vi "Teleop.vi"(10 "Match Info":T1={"Autonomous Elapsed Seconds"=0.0, "TeleOp Elapsed Seconds"=0.0, "Disabled Elapsed Seconds"=0.0, "Visited Autonomous"=FALSE, "Visited TeleOp"=FALSE, "Visited Disabled"=FALSE, "Autonomous Settings"={"Autonomous Style"=enum."Independent", "VI Refnum"=refnum}}, 11 "Call Context":T2) -> ()   [LabVIEW 2018]
doc: "This VI is called for each TeleOp packet received from the DS where the robot is not disabled. It is often used to read from the joysticks and update I/O or to update setpoints for timed control loops. It should complete and return within 20 milliseconds or it may miss DS packets."
uses:
  <vilib>/Rock Robotics/WPI/DriverStation/WPI_DriverStationDerivedRobotMode.ctl
  <vilib>/Rock Robotics/WPI/DriverStation/WPI_DriverStationMatch Info.ctl
  <vilib>/Rock Robotics/Network Tables/NT Read Boolean.vi
  <vilib>/Rock Robotics/Network Tables/NT Read Number.vi
  <vilib>/Rock Robotics/WPI/Utilities/WPI_GetSetVariantRefNum.vi
  <vilib>/Rock Robotics/Network Tables/NT Write Boolean Array.vi
  <vilib>/Rock Robotics/Network Tables/NT Write Numeric Array.vi
  <vilib>/Rock Robotics/Network Tables/NT Read Numeric Array.vi
  <vilib>/Rock Robotics/Network Tables/NT Write Boolean.vi
  <vilib>/Rock Robotics/Network Tables/NT Write Number.vi
panel:
  in  "Motor Stall":dbl format="%#_13g"
  out "Sample Slider 0":dbl(slide) scale=0.0..5.0
  out "Sample Boolean 1":bool
  out "Sample Boolean 0":bool
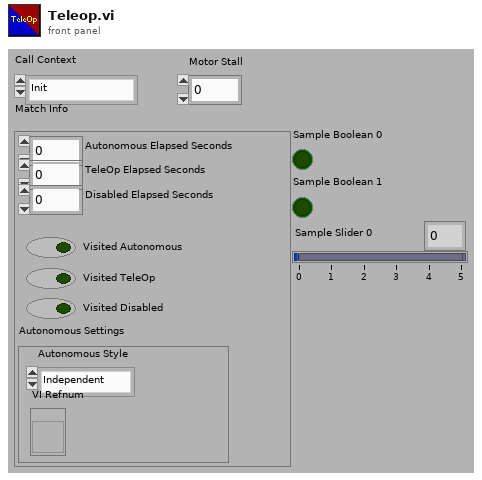
[diagram p1: front panel]
types:
  T1 = typedef "WPI_DriverStationMatch Info.ctl" = cluster{"Autonomous Elapsed Seconds":dbl, "TeleOp Elapsed Seconds":dbl, "Disabled Elapsed Seconds":dbl, "Visited Autonomous":bool, "Visited TeleOp":bool, "Visited Disabled":bool, "Autonomous Settings":cluster{"Autonomous Style":enum16{"Iterative", "Independent"}, "VI Refnum":refnum<vi>}}
  T2 = typedef "WPI_DriverStationDerivedRobotMode.ctl" = enum16{"Init", "Execute", "Stop"}
  T3 = typedef "WPI_JoystickDevRef.ctl" = cluster{"Device":T4}
  T4 = typedef "WPI_JoystickDeviceEnum.ctl" = enum16{"USB 0", "USB 1", "USB 2", "USB 3", "USB 4", "USB 5"}
  T5 = typedef "WPI_MotorControlDeviceRef.ctl" = cluster{"DeviceStatus":errorcluster, "Type":T6, "PWM":cluster{"PWM Channel":T7, "DeadBand":T8}, "CAN":cluster{"Device Number":u8, "SetOutput VI Ref":variant, "GetOutput VI Ref":variant, "Enable VI Ref":variant, "Disable VI Ref":variant, "Data":variant}, "Invert":bool, "DIO PWM":cluster{"PWM \"Enable\" Channel":T7, "DIOChannel":T9, "PWM Rate":dbl}}
  T6 = typedef "WPI_MotorControlType.ctl" = enum16{"PWM", "CAN", "DIO PWM"}
  T7 = typedef "FPGA_DIOPWMChannel.ctl" = enum8{"PWM 0", "PWM 1", "PWM 2", "PWM 3", "PWM 4", "PWM 5", "PWM 6", "PWM 7", "PWM 8", "PWM 9", "PWM MXP 0", "PWM MXP 1", "PWM MXP 2", "PWM MXP 3", "PWM MXP 4", "PWM MXP 5", "PWM MXP 6", "PWM MXP 7", "PWM MXP 8", "PWM MXP 9", "Invalid"}
  T8 = typedef "WPI_PWMDeadband.ctl" = cluster{"Name":string, "maxPositivePwm":i32, "minPositivePwm":i32, "centerPwm":i32, "maxNegativePwm":i32, "minNegativePwm":i32, "angularRange":u16}
  T9 = typedef "FPGA_DIOChannel.ctl" = enum8{"DIO 0", "DIO 1", "DIO 2", "DIO 3", "DIO 4", "DIO 5", "DIO 6", "DIO 7", "DIO 8", "DIO 9", "DIO MXP 0", "DIO MXP 1", "DIO MXP 2", "DIO MXP 3", "DIO MXP 4", "DIO MXP 5", "DIO MXP 6", "DIO MXP 7", "DIO MXP 8", "DIO MXP 9", "DIO MXP 10", "DIO MXP 11", "DIO MXP 12", "DIO MXP 13", "DIO MXP 14", "DIO MXP 15", "SPI Port CS1", "SPI Port CS2", "SPI Port CS3", "SPI Port MISO", "SPI Port MOSI", "Invalid"}
  T10 = typedef "WPI_RobotDriveDevRef.ctl" = cluster{"DevStatus":errorcluster, "Motors[]":T5[], "Square Inputs":bool, "Max Output":dbl}
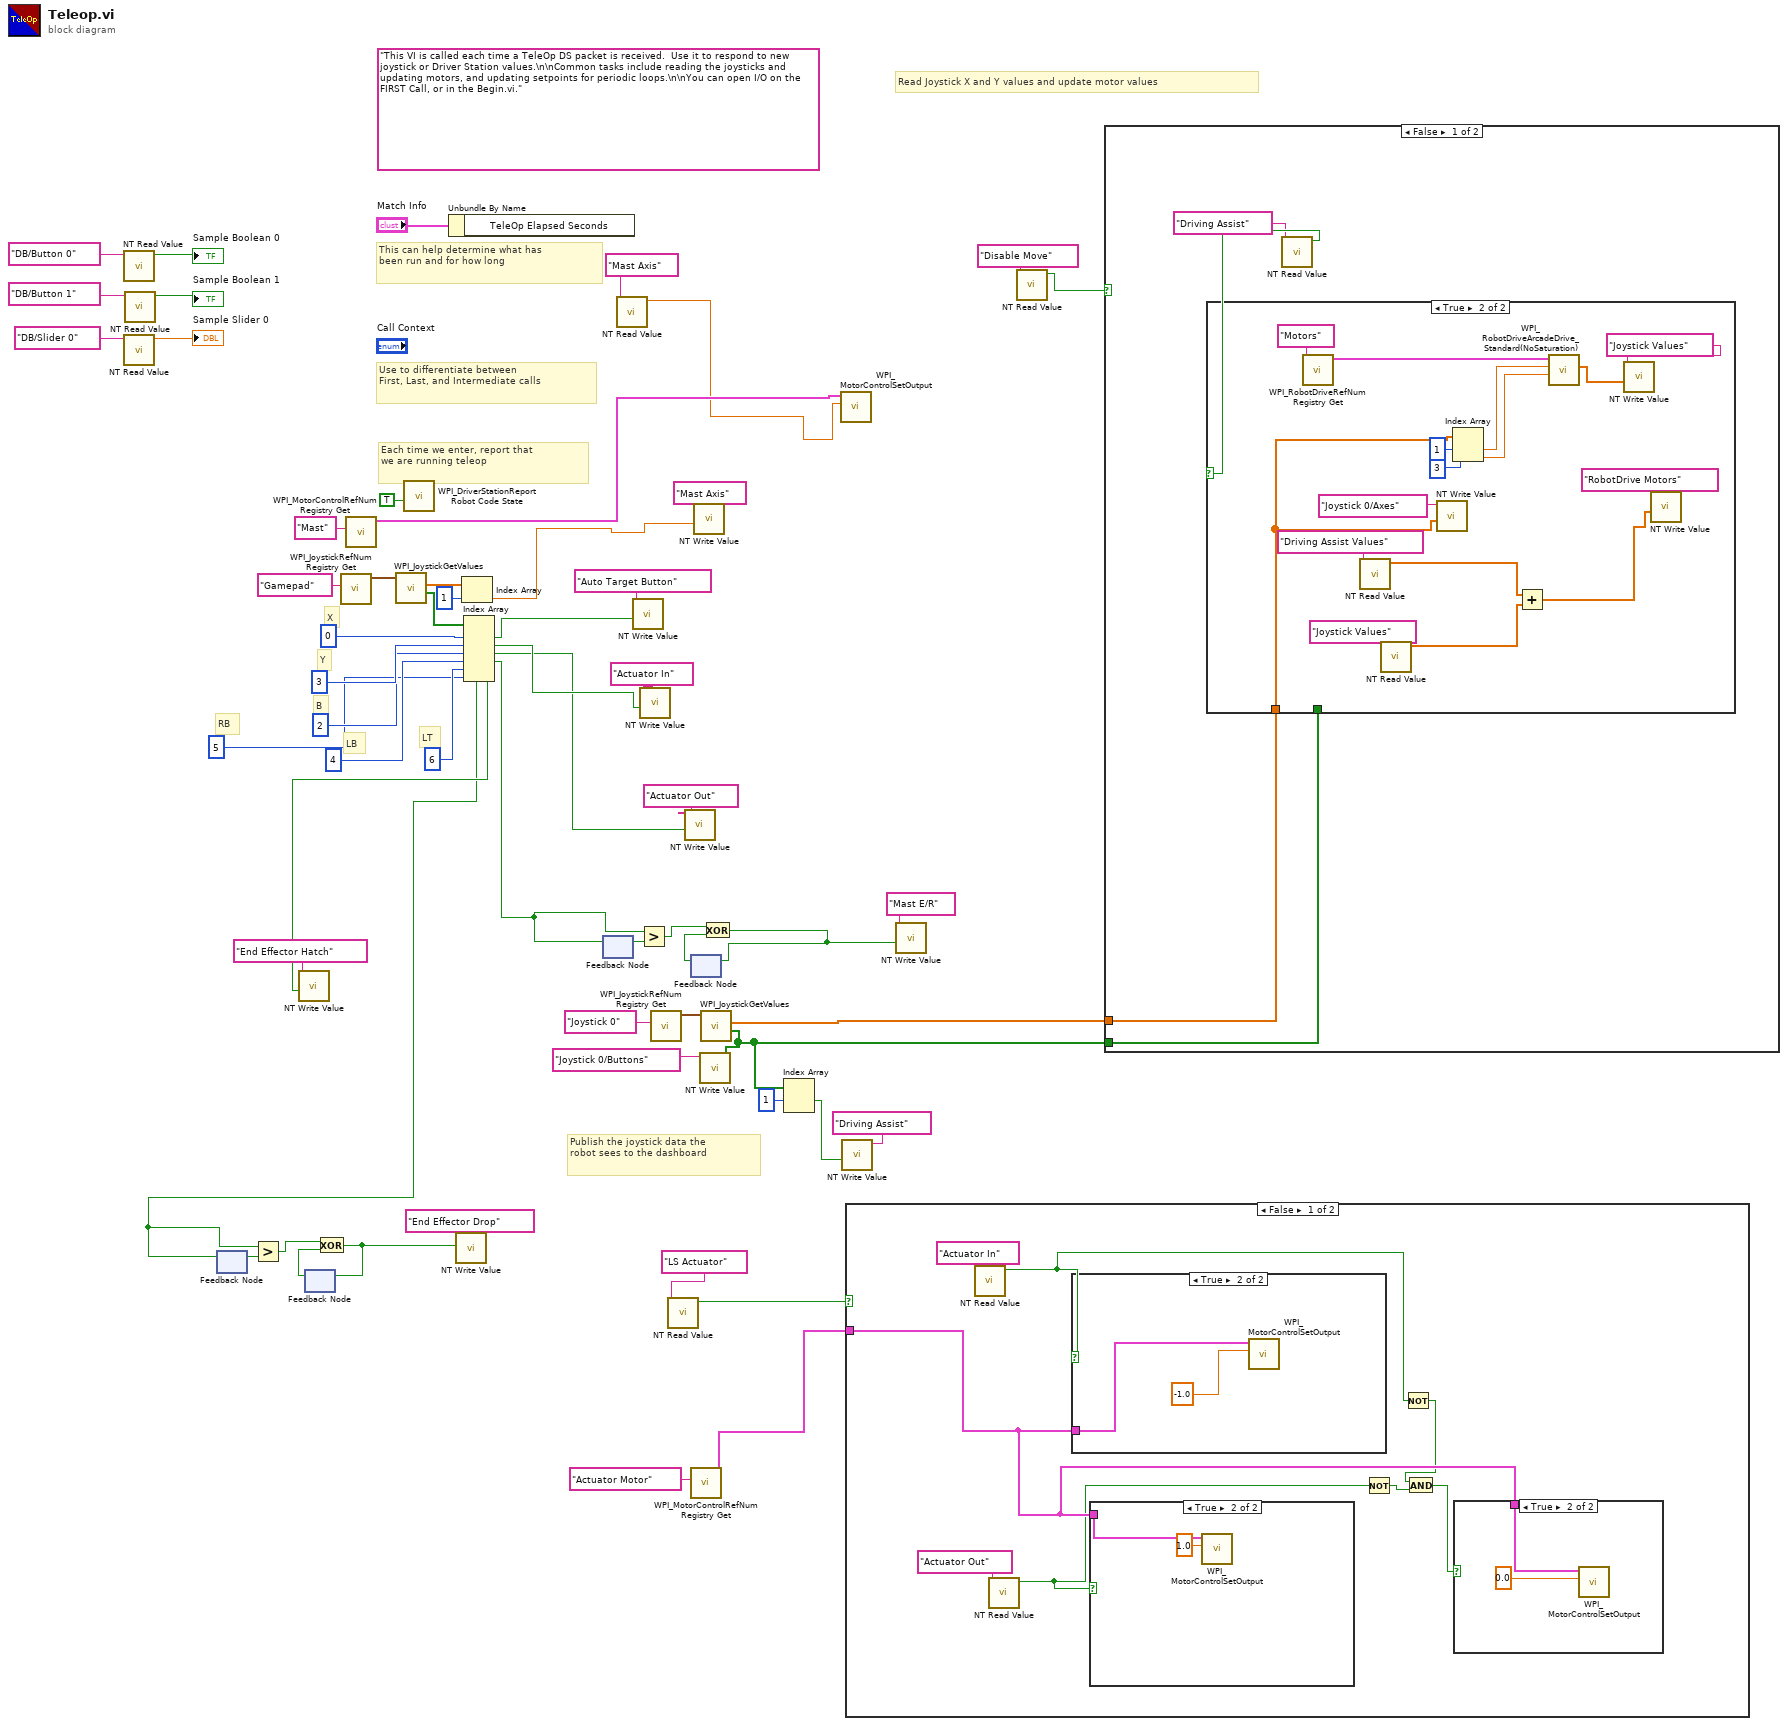
[diagram p0: block diagram]
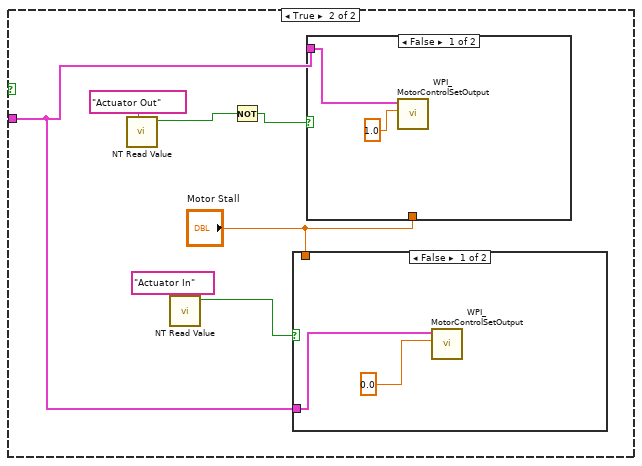
[diagram p5: hidden frame]
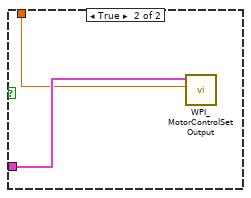
[diagram p6: hidden frame]
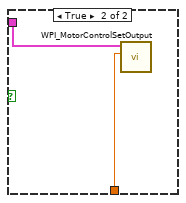
[diagram p7: hidden frame]
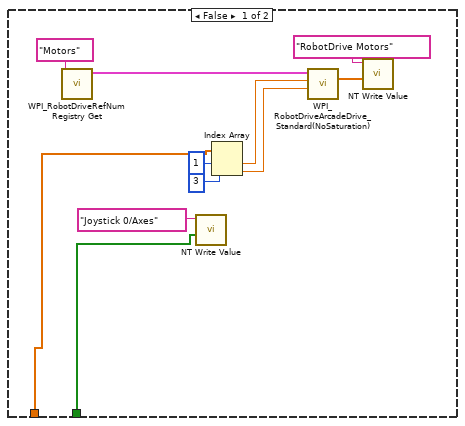
[diagram p8: hidden frame]
diagram:
  (unwired) "This VI is called each time a TeleOp DS packet is received.  Use it to respond to new joystick or Driver Station values.\n\nCommon tasks include reading the joysticks and updating motors, and updating setpoints for periodic loops.\n\nYou can open I/O on the FIRST Call, or in the Begin.vi."
  # "RB"
  # "LT"
  # "LB"
  # "Publish the joystick data the\nrobot sees to the dashboard"
  # "B"
  # "X"
  # "Y"
  # "Each time we enter, report that\nwe are running teleop"
  # "Use to differentiate between\nFirst, Last, and Intermediate calls"
  # "This can help determine what has\nbeen run and for how long"
  # "Read Joystick X and Y values and update motor values"
  n1 = call-poly <vilib>:"NT Read Value.vi"("Name"="DB/Button 0" ("refnum name")) -> ("Boolean"=→"Sample Boolean 0":bool)  [unwired: 9 in, 1 out]
  n2 = call-poly <vilib>:"NT Read Value.vi"("Name"="DB/Slider 0" ("refnum name")) -> ("Numeric"=→"Sample Slider 0":dbl)  [unwired: 9 in, 1 out]
  n3 = call-poly <vilib>:"NT Read Value.vi"("Name"="DB/Button 1" ("refnum name")) -> ("Boolean"=→"Sample Boolean 1":bool)  [unwired: 9 in, 1 out]
  n4 = feedback #1() -> (w5:bool)  [unwired: 1 in]
  n5 = feedback #2() -> (w3:bool)  [unwired: 1 in]
  n6 = call <vilib>:"WPI_JoystickRefNum Registry Get.vi"("refnum name"="Gamepad") -> ("JoystickDevRef"=w49:T3)  [unwired: 9 in, 1 out]
  n7 = call <vilib>:"WPI_MotorControlRefNum Registry Get.vi"("refnum name"="Mast") -> ("MotorControlDevRef"=w12:T5)  [unwired: 9 in, 1 out]
  n8 = call <vilib>:"WPI_JoystickGetValues.vi"("JoystickDevRef"=w49) -> ("Buttons"=w44:bool[], "Axes"=w48:dbl[])  [unwired: 6 in, 3 out]
  n9 = call <vilib>:"WPI_DriverStationReport Robot Code State.vi"("TeleOp"=TRUE ("Autonomous")) -> ()  [unwired: 10 in, 1 out]
  n10 = Unbundle By Name("Match Info") -> ()  [unwired: 1 out]
  n11 = Index Array(array=w48, index=1) -> (element=w15:dbl)
  n12 = Index Array(array=w44, index #1=0 ("index"), index #2=3 ("index"), index #3=2 ("index"), index #4=4 ("index"), index #5=6 ("index"), index #6=5 ("index")) -> (element #1=w42:bool, element #2=w36:bool, element #3=w33:bool, element #4=w10:bool, element #5=w2:bool, element #6=w20:bool)
  n13 = feedback-in #1(w2) -> ()
  n14 = Greater?(x=w2, y=w5) -> (0:w4:bool)
  n15 = call-poly <vilib>:"NT Write Value.vi"("Boolean"=w20, "Name"="End Effector Hatch") -> ()  [unwired: 9 in, 1 out]
  n16 = Exclusive Or(1:w3, 2:w4) -> (0:w1:bool)
  n17 = feedback-in #2(w1) -> ()
  n18 = call-poly <vilib>:"NT Write Value.vi"("Boolean"=w1, "Name"="End Effector Drop") -> ()  [unwired: 9 in, 1 out]
  n19 = feedback #3() -> (w9:bool)  [unwired: 1 in]
  n20 = feedback-in #3(w10) -> ()
  n21 = call-poly <vilib>:"NT Read Value.vi"("Name"="Mast Axis") -> ("Numeric"=w11:dbl)  [unwired: 9 in, 1 out]
  n22 = call-poly <vilib>:"NT Write Value.vi"("Boolean"=w42, "Name"="Auto Target Button") -> ()  [unwired: 9 in, 1 out]
  n23 = Greater?(x=w10, y=w9) -> (0:w8:bool)
  n24 = call-poly <vilib>:"NT Write Value.vi"("Boolean"=w36, "Name"="Actuator In") -> ()  [unwired: 9 in, 1 out]
  n25 = call <vilib>:"WPI_JoystickRefNum Registry Get.vi"("refnum name"="Joystick 0") -> ("JoystickDevRef"=w30:T3)  [unwired: 1 in, 9 out]
  n26 = call-poly <vilib>:"NT Read Value.vi"("Name"="LS Actuator") -> ("Boolean"=w39:bool)  [unwired: 9 in, 1 out]
  n27 = call-poly <vilib>:"NT Write Value.vi"("Boolean"=w33, "Name"="Actuator Out") -> ()  [unwired: 9 in, 1 out]
  n28 = feedback #4() -> (w6:bool)  [unwired: 1 in]
  n29 = call <vilib>:"WPI_MotorControlRefNum Registry Get.vi"("refnum name"="Actuator Motor") -> ("MotorControlDevRef"=w31:T5)  [unwired: 9 in, 1 out]
  n30 = call-poly <vilib>:"NT Write Value.vi"("Numeric"=w15, "Name"="Mast Axis") -> ()  [unwired: 9 in, 1 out]
  n31 = call <vilib>:"WPI_JoystickGetValues.vi"("JoystickDevRef"=w30) -> ("Buttons"=w26:bool[], "Axes"=w28:dbl[])  [unwired: 6 in, 3 out]
  n32 = call-poly <vilib>:"NT Write Value.vi"("Boolean Array"=w26, "Name"="Joystick 0/Buttons") -> ()  [unwired: 9 in, 1 out]
  n33 = Exclusive Or(1:w6, 2:w8) -> (0:w7:bool)
  n34 = feedback-in #4(w7) -> ()
  n35 = Index Array(array=w26, index #1=1 ("index")) -> (element #1=w24:bool)  [unwired: 1 in, 1 out]
  n36 = call <vilib>:"WPI_MotorControlSetOutput.vi"("Output"=w11, "MotorControlDevRef"=w12) -> ()  [unwired: 7 in, 3 out]
  n37 = call-poly <vilib>:"NT Write Value.vi"("Boolean"=w24, "Name"="Driving Assist") -> ()  [unwired: 9 in, 1 out]
  n38 = case shown="False" w39 {
    tunnel: w31 -> [w64 w75]
    frame False {
      n39 = call-poly <vilib>:"NT Read Value.vi"("Name"="Actuator In") -> ("Boolean"=w61:bool)  [unwired: 9 in, 1 out]
      n40 = call-poly <vilib>:"NT Read Value.vi"("Name"="Actuator Out") -> ("Boolean"=w62:bool)  [unwired: 9 in, 1 out]
      n41 = case shown="True" w61 {
        tunnel: w64 -> [_ w72]
        frame False {
        }
        frame True {
          n42 = call <vilib>:"WPI_MotorControlSetOutput.vi"("Output"=-1.0, "MotorControlDevRef"=w72) -> ()  [unwired: 7 in, 3 out]
        }
      }
      n43 = case shown="True" w62 {
        tunnel: w64 -> [_ w71]
        frame False {
        }
        frame True {
          n44 = call <vilib>:"WPI_MotorControlSetOutput.vi"("Output"=1.0, "MotorControlDevRef"=w71) -> ()  [unwired: 7 in, 3 out]
        }
      }
      n45 = Not(x=w62) -> (.not. x?=w63:bool)
      n46 = Not(x=w61) -> (.not. x?=w60:bool)
      n47 = And(x=w60, y=w63) -> (x .and. y?=w65:bool)
      n48 = case shown="True" w65 {
        tunnel: w64 -> [_ w68]
        frame False {
        }
        frame True {
          n49 = call <vilib>:"WPI_MotorControlSetOutput.vi"("Output"=0.0, "MotorControlDevRef"=w68) -> ()  [unwired: 7 in, 3 out]
        }
      }
    }
    frame True {
      n50 = call-poly <vilib>:"NT Read Value.vi"("Name"="Actuator Out") -> ("Boolean"=w79:bool)  [unwired: 9 in, 1 out]
      n51 = call-poly <vilib>:"NT Read Value.vi"("Name"="Actuator In") -> ("Boolean"=w76:bool)  [unwired: 9 in, 1 out]
      n52 = Not(x=w79) -> (.not. x?=w78:bool)
      n53 = case shown="False" w76 {
        tunnel: w75 -> [w81 w84]
        tunnel: "Motor Stall" -> [_ w83]
        frame False {
          n54 = call <vilib>:"WPI_MotorControlSetOutput.vi"("Output"=0.0, "MotorControlDevRef"=w81) -> ()  [unwired: 7 in, 3 out]
        }
        frame True {
          n55 = call <vilib>:"WPI_MotorControlSetOutput.vi"("Output"=w83, "MotorControlDevRef"=w84) -> ()  [unwired: 7 in, 3 out]
        }
      }
      n56 = case shown="False" w78 {
        tunnel: w75 -> [w86 w88]
        tunnel: "Motor Stall" -> [_ w87]
        frame False {
          n57 = call <vilib>:"WPI_MotorControlSetOutput.vi"("Output"=1.0, "MotorControlDevRef"=w86) -> ()  [unwired: 7 in, 3 out]
        }
        frame True {
          n58 = call <vilib>:"WPI_MotorControlSetOutput.vi"("Output"=w87, "MotorControlDevRef"=w88) -> ()  [unwired: 7 in, 3 out]
        }
      }
    }
  }
  n59 = call-poly <vilib>:"NT Write Value.vi"("Boolean"=w7, "Name"="Mast E/R") -> ()  [unwired: 9 in, 1 out]
  n60 = call-poly <vilib>:"NT Read Value.vi"("Name"="Disable Move") -> ("Boolean"=w46:bool)  [unwired: 9 in, 1 out]
  n61 = case shown="False" w46 {
    tunnel: w26 -> [w91 _]
    tunnel: w28 -> [w92 _]
    frame False {
      n62 = call-poly <vilib>:"NT Read Value.vi"("Name"="Driving Assist") -> ("Boolean"=w90:bool)  [unwired: 9 in, 1 out]
      n63 = case shown="True" w90 {
        tunnel: w92 -> [w94 w112]
        tunnel: w91 -> [w93 _]
        frame False {
          n64 = call <vilib>:"WPI_RobotDriveRefNum Registry Get.vi"("refnum name"="Motors") -> ("RobotDriveDevRef"=w102:T10)  [unwired: 1 in, 9 out]
          n65 = call-poly <vilib>:"NT Write Value.vi"("Boolean Array"=w93, "Name"="Joystick 0/Axes") -> ()  [unwired: 9 in, 1 out]
          n66 = Index Array(array=w94, index #1=1 ("index"), index #2=3 ("index")) -> (element #1=w101:dbl, element #2=w100:dbl)
          n67 = call <vilib>:"WPI_RobotDriveArcadeDrive_Standard(NoSaturation).vi"("Y axis value"=w100, "X axis value"=w101, "RobotDriveDevRef"=w102) -> ("Motor Values"=w98:dbl[])  [unwired: 1 in, 7 out]
          n68 = call-poly <vilib>:"NT Write Value.vi"("Numeric Array"=w98, "Name"="RobotDrive Motors") -> ()  [unwired: 9 in, 1 out]
        }
        frame True {
          n69 = call <vilib>:"WPI_RobotDriveRefNum Registry Get.vi"("refnum name"="Motors") -> ("RobotDriveDevRef"=w118:T10)  [unwired: 1 in, 9 out]
          n70 = call-poly <vilib>:"NT Read Value.vi"("Name"="Driving Assist Values") -> ("Numeric Array"=w107:dbl[])  [unwired: 9 in, 1 out]
          n71 = call-poly <vilib>:"NT Read Value.vi"("Name"="Joystick Values") -> ("Numeric Array"=w106:dbl[])  [unwired: 9 in, 1 out]
          n72 = call-poly <vilib>:"NT Write Value.vi"("Numeric Array"=w112, "Name"="Joystick 0/Axes") -> ()  [unwired: 9 in, 1 out]
          n73 = Index Array(array=w112, index #1=1 ("index"), index #2=3 ("index")) -> (element #1=w117:dbl, element #2=w116:dbl)
          n74 = Add(x=w107, y=w106) -> (x+y=w104:dbl[])
          n75 = call <vilib>:"WPI_RobotDriveArcadeDrive_Standard(NoSaturation).vi"("Y axis value"=w116, "X axis value"=w117, "RobotDriveDevRef"=w118) -> ("Motor Values"=w110:dbl[])  [unwired: 1 in, 7 out]
          n76 = call-poly <vilib>:"NT Write Value.vi"("Numeric Array"=w110, "Name"="Joystick Values") -> ()  [unwired: 9 in, 1 out]
          n77 = call-poly <vilib>:"NT Write Value.vi"("Numeric Array"=w104, "Name"="RobotDrive Motors") -> ()  [unwired: 9 in, 1 out]
        }
      }
    }
    frame True {
    }
  }
